vi "Read_Write_Calibrations.vi"(6 "Silent?":bool, 7 "Task":enum16{"Save", "Read", "List"}(ring)=enum."Read", 9 "Calibration name":string="Default", 11 "Settings in":T1={"Name of test"="", "Date"=timestamp(0 s since 1904-01-01), "Location"="", "Template"="", "Soundcard"="", "resolution"=32, "Sampling rate"=48000, "Ch1 Gain "=25.0, "Ch2 Gain"=10.0, "Sample time (s)"=0.3, "Pre-trigger (s)"=0.01, "Hammer Threshold"=10.0, "Positions"=12, "Taps/Position"=5, "Set Names"="", "Freq resolution"=10.0, "Hammer cutoff"=0.0, "Mic cutoff"=0.0, "Double bounce "=0.0, "Hammer Cal"=10.0, "dB Offset"=0.0, "Accel Cal"=10.0, "Vibrometer Cal"=0.0, "Mic Cal"=0.0, "Output"=2, "Voltage Cal"=1.0, "Vibrometer Port"="ASRL27::INSTR", "Range"=4, "High Pass"=2, "Bandwidth"=4, "X Range"=[], "Y Range"=[], "dB Spread"=0.0, "Trigger"=0, "Ch_1"=25, "Ch_2"=25, "flip?"=FALSE, "60Hz"=FALSE, "Time offset"=0.0, "Piezo Cal"=1.0, "Default Notes"=""} {"Ch_2" min=1 step=1; "Ch_1" min=1 max=100 step=1; "Trigger" items=["Hammer (force)", "Self-tap", "Spacebar"]; "Bandwidth" items=["1 kHz"=1, "5 kHz"=5, "10 kHz"=10, "25 kHz"=25, "50 kHz"=50, "100 kHz"=100]; "High Pass" items=["Off", "13 Hz", "104 Hz"]; "Range" items=["10 mm/s"=1, "20 mm/s"=2, "50 mm/s"=5, "100 mm/s"=10, "200 mm/s"=20, "500 mm/s"=50, "1 m/s"=100, "2 m/s"=200]; "Output" items=["Accelerometer", "Speed (from acceleration)", "Microphone", "Vibrometer", "Piezo"]; "Voltage Cal" format="%#_13g"; "Ch2 Gain" format="%#_13g"; "Ch1 Gain" format="%#_13g"; "Double bounce" min=0.0; "Mic cutoff" min=0.0 format="%#_4g"; "Hammer cutoff" min=0.0 format="%#_4g"; "Freq resolution" min=0.0; "Pre-trigger (s)" format="%#_13g"; "Date" format="%<%H:%M\n%d/%m/%y>T"; "resolution" items=["16 bit"=16, "24 bit"=24, "32 bit"=32]; "Sampling rate" items=["22050 samp/s"=22050, "44100 samp/s"=44100, "48000 samp/s"=48000]}) -> (0 "file":string, 1 "Cal files":string[](array[string]), 3 "Settings out":T1={"Name of test"="", "Date"=timestamp(0 s since 1904-01-01), "Location"="", "Template"="", "Soundcard"="", "resolution"=32, "Sampling rate"=48000, "Ch1 Gain "=25.0, "Ch2 Gain"=10.0, "Sample time (s)"=0.3, "Pre-trigger (s)"=0.01, "Hammer Threshold"=10.0, "Positions"=12, "Taps/Position"=5, "Set Names"="", "Freq resolution"=10.0, "Hammer cutoff"=0.0, "Mic cutoff"=0.0, "Double bounce "=0.0, "Hammer Cal"=10.0, "dB Offset"=0.0, "Accel Cal"=10.0, "Vibrometer Cal"=0.0, "Mic Cal"=0.0, "Output"=2, "Voltage Cal"=1.0, "Vibrometer Port"="ASRL27::INSTR", "Range"=4, "High Pass"=2, "Bandwidth"=4, "X Range"=[], "Y Range"=[], "dB Spread"=0.0, "Trigger"=0, "Ch_1"=25, "Ch_2"=25, "flip?"=FALSE, "60Hz"=FALSE, "Time offset"=0.0, "Piezo Cal"=1.0, "Default Notes"=""} {"Ch_2" min=1 step=1; "Ch_1" min=1 max=100 step=1; "Trigger" items=["Hammer (force)", "Self-tap", "Spacebar"]; "Bandwidth" items=["1 kHz"=1, "5 kHz"=5, "10 kHz"=10, "25 kHz"=25, "50 kHz"=50, "100 kHz"=100]; "High Pass" items=["Off", "13 Hz", "104 Hz"]; "Range" items=["10 mm/s"=1, "20 mm/s"=2, "50 mm/s"=5, "100 mm/s"=10, "200 mm/s"=20, "500 mm/s"=50, "1 m/s"=100, "2 m/s"=200]; "Output" items=["Accelerometer", "Speed (from acceleration)", "Microphone", "Vibrometer", "Piezo"]; "Voltage Cal" format="%#_13g"; "Ch2 Gain" format="%#_13g"; "Ch1 Gain" format="%#_13g"; "Double bounce" min=0.0; "Mic cutoff" min=0.0 format="%#_4g"; "Hammer cutoff" min=0.0 format="%#_4g"; "Freq resolution" min=0.0; "Pre-trigger (s)" format="%#_13g"; "Date" format="%<%H:%M\n%d/%m/%y>T"; "resolution" items=["16 bit"=16, "24 bit"=24, "32 bit"=32]; "Sampling rate" items=["22050 samp/s"=22050, "44100 samp/s"=44100, "48000 samp/s"=48000]})   [LabVIEW 2022 SP3]
uses:
  PreferencesControl.ctl
panel:
  out "Path to Calibrations":path
  out "error out":errorcluster
  in  "error in":errorcluster
  # "Hz"
  # "dB"
  # "dB"
  # "sec"
  # "sec"
  # "mV/Pa"
  # "mV/m/s2"
  # "mV/mm/s"
  # "V/N"
  # "sec"
  # "sec"
  # "mV/N"
  # "a.u."
  # "a.u."
  # "sec"
  # "Hz"
  # "dB"
  # "dB"
  # "sec"
  # "sec"
  # "mV/Pa"
  # "mV/m/s2"
  # "mV/mm/s"
  # "V/N"
  # "sec"
  # "sec"
  # "mV/N"
  # "a.u."
  # "a.u."
  # "sec"
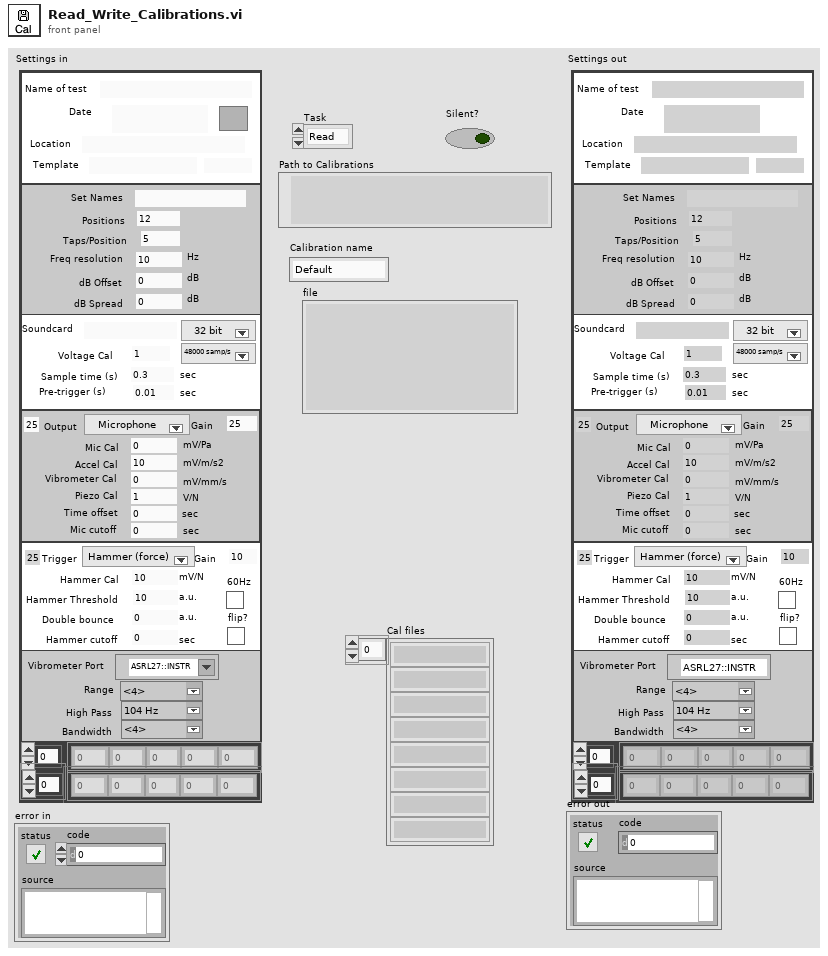
[diagram p1: front panel]
types:
  T1 = typedef "PreferencesControl.ctl" = cluster{"Name of test":string, "Date":timestamp, "Location":string, "Template":string, "Soundcard":string, "resolution":u16, "Sampling rate":u16, "Ch1 Gain ":dbl, "Ch2 Gain":dbl, "Sample time (s)":dbl, "Pre-trigger (s)":dbl, "Hammer Threshold":dbl, "Positions":i16, "Taps/Position":i16, "Set Names":string, "Freq resolution":dbl, "Hammer cutoff":dbl, "Mic cutoff":dbl, "Double bounce ":dbl, "Hammer Cal":dbl, "dB Offset":dbl, "Accel Cal":dbl, "Vibrometer Cal":dbl, "Mic Cal":dbl, "Output":u16, "Voltage Cal":dbl, "Vibrometer Port":refnum<visa-resource-name>, "Range":u16, "High Pass":u16, "Bandwidth":u16, "X Range":cluster{"Minimum":dbl, "Maximum":dbl, "Increment":dbl, "Minor Increment":dbl, "Start":dbl}[], "Y Range":cluster{"Minimum":dbl, "Maximum":dbl, "Increment":dbl, "Minor Increment":dbl, "Start":dbl}[], "dB Spread":dbl, "Trigger":u16, "Ch_1":u8, "Ch_2":u8, "flip?":bool, "60Hz":bool, "Time offset":dbl, "Piezo Cal":dbl, "Default Notes":string}
  T2 = cluster{"Voltage Cal":dbl, "Mic Cal":dbl, "Accel Cal":dbl, "Vibrometer Cal":dbl, "Hammer Cal":dbl, "Piezo Cal":dbl, "flip":dbl}
  T3 = cluster{"[0]":dbl, "[1]":dbl, "[2]":dbl, "[3]":dbl, "[4]":dbl, "[5]":dbl, "[6]":dbl}
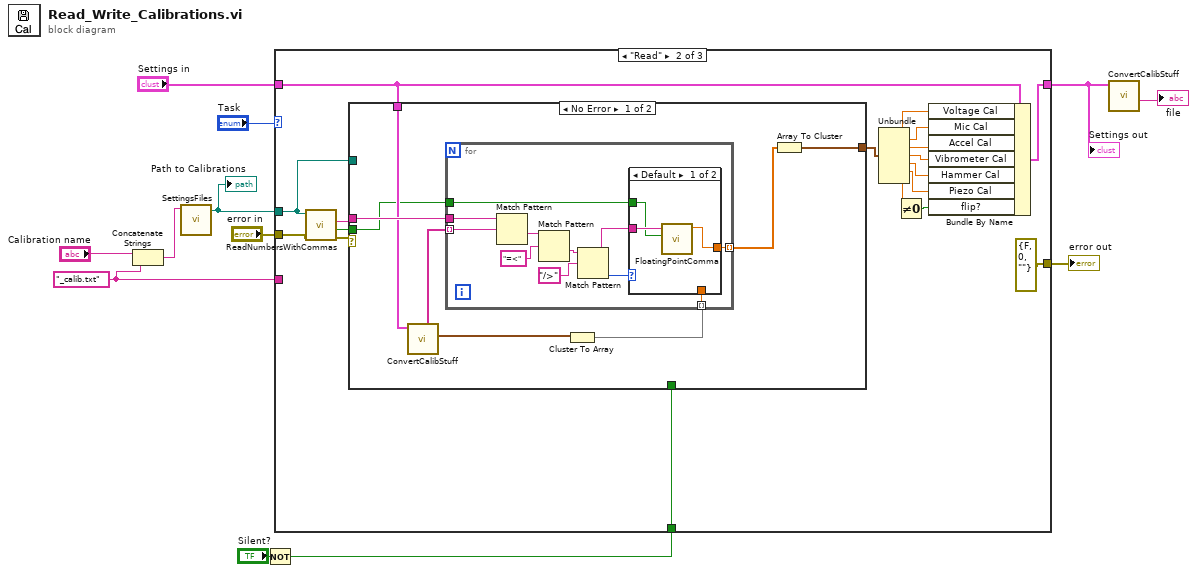
[diagram p0: block diagram]
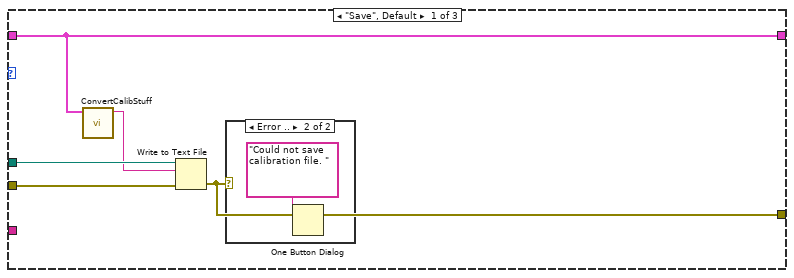
[diagram p2: hidden frame]
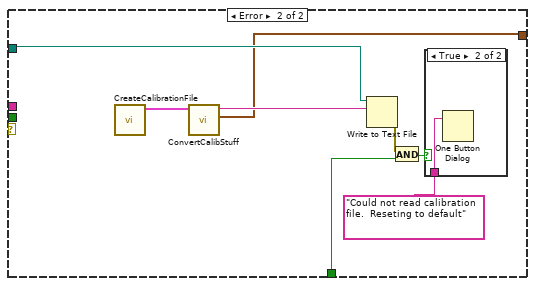
[diagram p5: hidden frame]
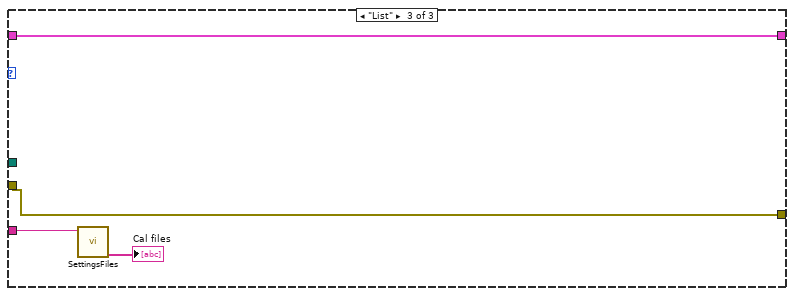
[diagram p7: hidden frame]
diagram:
  w1 = "_calib.txt" ("name or relative path")
  n1 = Concatenate Strings("Calibration name", w1) -> (w3:string)
  n2 = call "SettingsFiles.vi"("settings file name"=w3) -> ("file path"=w2:path)  [unwired: 9 in, 1 out]
  "Path to Calibrations" <- w2
  n3 = Not(x="Silent?") -> (.not. x?=w6:bool)
  n4 = case shown="\"Read\"" "Task" {
    tunnel: w2 -> [w16 w24 _]
    tunnel: "error in" -> [w15 w23 w69]
    tunnel: "Settings in" -> [w17 w27 w72]
    tunnel: [w17 w30 w72] -> w5
    tunnel: [w13 errorcluster {"status"=FALSE, "code"=0, "source"=""} ("error out") w69] -> w9
    tunnel: w1 -> [_ _ w70]
    tunnel: w6 -> [_ w28 _]
    frame "Save", Default {
      n5 = call "ConvertCalibStuff.vi"("Settings in"=w17) -> ("File"=w14:string)  [unwired: 7 in, 3 out]
      n6 = Write to Text File(file (use dialog)=w16, text=w14, error in=w15) -> (error out=w13:errorcluster)  [unwired: 1 in, 2 out]
      n7 = case shown="Error .." w13 {
        frame No Error {
        }
        frame Error {
          n8 = One Button Dialog(message="Could not save calibration file. ") -> ()  [unwired: 1 in, 1 out]
        }
      }
    }
    frame "Read" {
      n9 = call "ReadNumbersWithCommas.vi"("error in"=w23, "file (use dialog)"=w24) -> ("error out"=w26:errorcluster, "comma?"=w22:bool, "text"=w25:string)  [unwired: 6 in, 1 out]
      n10 = case shown="No Error" w26 {
        tunnel: w25 -> [w44 _]
        tunnel: [w42 w60] -> w36
        tunnel: w24 -> [_ w67]
        tunnel: w28 -> [_ w64]
        tunnel: w27 -> [w40 _]
        tunnel: w22 -> [w37 _]
        frame No Error {
          n11 = call "ConvertCalibStuff.vi"("Settings in"=w40) -> ("cluster"=w39:T2, "titles"=w38:string[])  [unwired: 7 in, 2 out]
          n12 = Cluster To Array(cluster=w39) -> (array=w41:dbl[])
          n13 = for {
            tunnel: w44 -> [w51]
            tunnel: [w48] -> w43 mode=indexing
            tunnel: w41 -> [w47] mode=indexing
            tunnel: w38 -> [w46] mode=indexing
            tunnel: w37 -> [w45]
            n14 = Match Pattern(string=w51, regular expression=w46) -> (after substring=w52:string)  [unwired: 1 in, 3 out]
            n15 = Match Pattern(string=w52, regular expression="=<" ("format string")) -> (after substring=w53:string)  [unwired: 1 in, 3 out]
            n16 = Match Pattern(string=w53, regular expression="/>" ("format string")) -> (before substring=w49:string, offset past match=w50:i32)  [unwired: 1 in, 2 out]
            n17 = case shown="Default" w50 {
              tunnel: w49 -> [w58 _]
              tunnel: [w57 w59] -> w48
              tunnel: w47 -> [_ w59]
              tunnel: w45 -> [w56 _]
              frame Default {
                n18 = call "FloatingPointComma.vi"("Comma?"=w56, "String In"=w58) -> ("Numeric"=w57:dbl)  [unwired: 8 in, 1 out]
              }
              frame -1 {
              }
            }
          }
          n19 = Array To Cluster(array=w43) -> (cluster=w42:T3)
        }
        frame Error {
          n20 = call "CreateCalibrationFile.vi"() -> ("Settings out"=w62:T1)  [unwired: 11 in]
          n21 = call "ConvertCalibStuff.vi"("Settings in"=w62) -> ("cluster"=w60:T2, "File"=w61:string)  [unwired: 7 in, 2 out]
          n22 = Write to Text File(file (use dialog)=w67, text=w61) -> (error out=w65:errorcluster)  [unwired: 2 in, 2 out]
          n23 = And(x=w65, y=w64) -> (x .and. y?=w63:bool)
          n24 = case shown="True" w63 {
            tunnel: "Could not read calibration file.  Reseting to default" ("message") -> [_ w68]
            frame False {
            }
            frame True {
              n25 = One Button Dialog(message=w68) -> ()  [unwired: 1 in, 1 out]
            }
          }
        }
      }
      n26 = Unbundle(w36) -> ("Voltage Cal"=w35:dbl, "Mic Cal"=w34:dbl, "Accel Cal"=w33:dbl, "Vibrometer Cal"=w32:dbl, "Hammer Cal"=w31:dbl, "Piezo Cal"=w21:dbl, "flip"=w19:dbl)
      n27 = Not Equal To 0?(x=w19) -> (x != 0?=w20:bool)
      n28 = Bundle By Name(cluster=w27, "Voltage Cal"=w35, "Mic Cal"=w34, "Accel Cal"=w33, "Vibrometer Cal"=w32, "Hammer Cal"=w31, "Piezo Cal"=w21, "flip?"=w20) -> (w30:T1)
    }
    frame "List" {
      n29 = call "SettingsFiles.vi"("settings file name"=w70) -> ("filenames"=→"Cal files":string[])  [unwired: 9 in, 1 out]
    }
  }
  "Settings out" <- w5
  "error out" <- w9
  n30 = call "ConvertCalibStuff.vi"("Settings in"=w5) -> ("Text"=→"file":string)  [unwired: 7 in, 3 out]
